vi "Add Monitor Queue Status Section.vi"(8 "error in":errorcluster, 11 "Custom Device Ref in":T1 format="%.0x") -> (0 "error out":errorcluster, 1 "Monitor Queue Status channel Refs":T1[](array[typedef]) format="%.0x", 2 "Monitor Queue Status Section Ref out":T1 format="%.0x", 3 "Custom Device Ref out":T1 format="%.0x")   [LabVIEW 2020, in "afdx_custom_device Scripting.lvlib"]
uses:
  afdx_custom_device Scripting.lvlib
  <vilib>/NI VeriStand/Custom Device API/Custom Device Item Ref.ctl
  <vilib>/NI VeriStand/Custom Device API/Custom Device Channel.ctl
  <vilib>/NI VeriStand/Custom Device API/Custom Device Channel Type.ctl
  Constants.vi
  <vilib>/NI VeriStand/Custom Device API/Custom Device API.lvlib
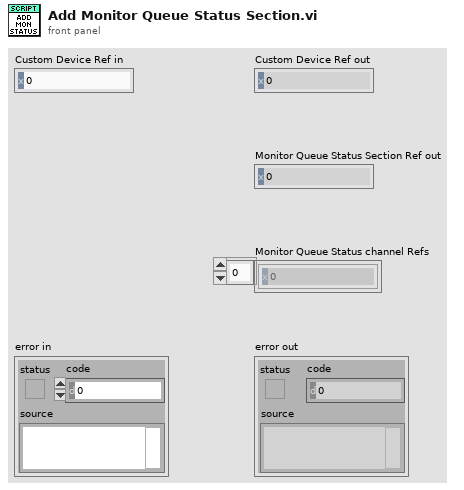
[diagram p1: front panel]
types:
  T1 = typedef "Custom Device API.lvlib/Custom Device Item Ref.ctl" = u64
  T2 = typedef "Custom Device API.lvlib/Custom Device Channel.ctl" = cluster{"Type":T3, "Units":string, "Default Value":dbl, "Faultable":bool, "Scalable":bool}
  T3 = typedef "Custom Device API.lvlib/Custom Device Channel Type.ctl" = enum16{"Input", "Output"}
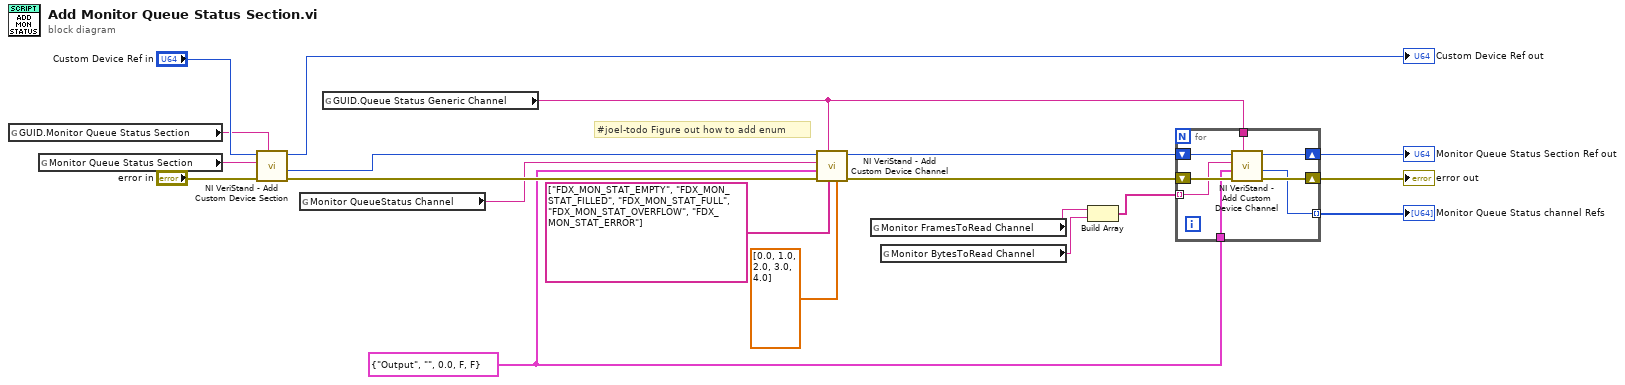
[diagram p0: block diagram]
diagram:
  w3 = T2 {"Type"=enum."Output", "Units"="", "Default Value"=0.0, "Faultable"=FALSE, "Scalable"=FALSE} ("Channel")
  # "#joel-todo Figure out how to add enum"
  n1 = global read "Constants.vi" "GUID.Monitor Queue Status Section"() -> (w16:string)
  n2 = global read "Constants.vi" "Monitor Queue Status Section"() -> (w18:string)
  n3 = call <vilib>:"NI VeriStand - Add Custom Device Section.vi"("GUID (Default Section)"=w16, "error in (no error)"="error in", "Section Name"=w18, "Parent Ref in"="Custom Device Ref in") -> ("error out"=w17:errorcluster, "Section Ptr"=w7:T1, "Parent Ref out"=→"Custom Device Ref out":T1)  [unwired: 4 in, 1 out]
  n4 = global read "Constants.vi" "Monitor QueueStatus Channel"() -> (w4:string)
  n5 = global read "Constants.vi" "GUID.Queue Status Generic Channel"() -> (w5:string)
  n6 = call <vilib>:"NI VeriStand - Add Custom Device Channel.vi"("Property Values"=dbl[] [0.0, 1.0, 2.0, 3.0, 4.0], "Property names"=string[] ["FDX_MON_STAT_EMPTY", "FDX_MON_STAT_FILLED", "FDX_MON_STAT_FULL", "FDX_MON_STAT_OVERFLOW", "FDX_MON_STAT_ERROR"], "GUID (Default Channel)"=w5, "error in (no error)"=w17, "Channel"=w3, "Channel Name"=w4, "Parent Ref in"=w7) -> ("error out"=w8:errorcluster, "Parent Ref out"=w6:T1)  [unwired: 1 in, 2 out]
  n7 = global read "Constants.vi" "Monitor FramesToRead Channel"() -> (w11:string)
  n8 = global read "Constants.vi" "Monitor BytesToRead Channel"() -> (w10:string)
  n9 = Build Array(w11, w10) -> (w9:string[])
  n10 = for {
    tunnel: [w24] -> w12 mode=indexing
    shift-right: [w25] -> w13
    shift-left: w8 -> [w28]
    tunnel: w9 -> [w23] mode=indexing
    tunnel: w3 -> [w22]
    tunnel: w5 -> [w21]
    shift-right: [w27] -> w15
    shift-left: w6 -> [w26]
    n11 = call <vilib>:"NI VeriStand - Add Custom Device Channel.vi"("GUID (Default Channel)"=w21, "error in (no error)"=w28, "Channel"=w22, "Channel Name"=w23, "Parent Ref in"=w26) -> ("error out"=w25:errorcluster, "Channel Ref"=w24:T1, "Parent Ref out"=w27:T1)  [unwired: 3 in, 1 out]
  }
  "Monitor Queue Status Section Ref out" <- w15
  "error out" <- w13
  "Monitor Queue Status channel Refs" <- w12
